vi "TEST.vi"() -> ()   [LabVIEW 2024]
panel:
  in  "Color Box":u32(colorbox)
  in  "Radio Buttons":enum32{"Radio Selection 1", "Radio Selection 2"}(radio)
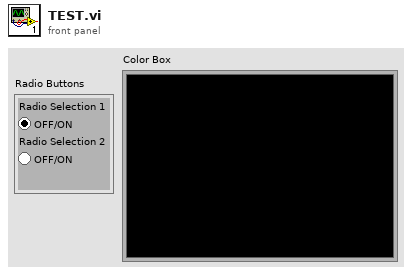
[diagram p1: front panel]
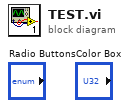
[diagram p0: block diagram]
diagram:
